vi "Rio_Trapazodial_Velocity_V2.vi"() -> ()   [LabVIEW 2017]
uses:
  <vilib>/myRIO/Common/Instrument Driver Framework/myRIO v1.0/Encoder/typedefs/Encoder Signal Mode.ctl
  <vilib>/myRIO/Instrument Drivers/Onboard IO/Encoder/typedefs/Encoder Reference.ctl
  <vilib>/myRIO/Common/Instrument Driver Framework/Utilities/typedefs/myRIO Generic Hardware Reference.ctl
  <vilib>/myRIO/Common/Instrument Driver Framework/Utilities/typedefs/Hardware Version Enum.ctl
  <vilib>/myRIO/Common/Instrument Driver Framework/Utilities/typedefs/myRIO v1.0 Reference.ctl
  <vilib>/myRIO/Common/Instrument Driver Framework/Utilities/typedefs/Generic FPGA Reference.ctl
  <vilib>/myRIO/Common/Instrument Driver Framework/myRIO v1.0/Encoder/typedefs/Encoder Channels Enum.ctl
  <vilib>/myRIO/Common/Instrument Driver Framework/myRIO v1.0/Encoder/typedefs/Encoder Configuration v1.0.ctl
  <vilib>/userdefined/High Color/nirio_resource_hc.ctl
  <vilib>/myRIO/Common/Instrument Driver Framework/Utilities/vis/Is FPGA Ref Available.vi
  <vilib>/myRIO/Common/Instrument Driver Framework/myRIO v1.0/Encoder/vis/myRIO v1.1 Open Encoder.vi
  <vilib>/myRIO/Instrument Drivers/Onboard IO/Encoder/vis/Read.vi
  <vilib>/myRIO/Common/Instrument Driver Framework/Utilities/vis/Validate Channels.vi
  <vilib>/myRIO/Common/Instrument Driver Framework/myRIO v1.0/Encoder/vis/myRIO v1.0 Reserve Encoder.vi
  <vilib>/myRIO/Common/Instrument Driver Framework/myRIO v1.0/Encoder/vis/myRIO v1.0 Build MUX Configuration Encoder.vi
  <vilib>/myRIO/Common/Instrument Driver Framework/myRIO v1.0/Resource Manager/vis/myRIO v1.0 Reserve Channel List.vi
  <vilib>/myRIO/Common/Instrument Driver Framework/myRIO v1.0/Resource Manager/vis/myRIO v1.0 Create Configuration List.vi
  <vilib>/myRIO/Common/Instrument Driver Framework/myRIO v1.0/Resource Manager/vis/myRIO v1.0 Reserve Channel.vi
  <vilib>/myRIO/Common/Instrument Driver Framework/myRIO v1.0/Resource Manager/vis/myRIO v1.0 Unreserve Channel.vi
  <vilib>/myRIO/Common/Instrument Driver Framework/myRIO v1.0/Resource Manager/vis/myRIO v1.0 Build Mutex Name.vi
  <vilib>/Utility/VariantDataType/GetNumericInfo.vi
  <vilib>/Utility/error.llb/Error Cluster From Error Code.vi
  <vilib>/myRIO/Common/Instrument Driver Framework/myRIO v1.0/myRIO v1.1 Open.vi
  <vilib>/myRIO/Common/Instrument Driver Framework/Utilities/vis/IO Manager.vi
  <vilib>/myRIO/Common/Instrument Driver Framework/Utilities/vis/Configuration Manager.vi
  <vilib>/myRIO/Common/Instrument Driver Framework/myRIO v1.0/Resource Manager/vis/myRIO v1.0 Configure IO.vi
  <vilib>/myRIO/Common/Instrument Driver Framework/myRIO v1.0/myRIO v1.0 Close.vi
  <vilib>/myRIO/Common/Instrument Driver Framework/myRIO v1.0/Encoder/vis/myRIO v1.0 Configure Encoder.vi
  <vilib>/myRIO/Common/Instrument Driver Framework/myRIO v1.0/Encoder/vis/myRIO v1.0 Read Encoder.vi
  <vilib>/addons/control/pid/pid.llb/PID (DBL).vi
  <vilib>/myRIO/Express VI/Onboard IO/Encoder/Encoder Express VI.xnode
  <vilib>/myRIO/Instrument Drivers/Onboard IO/Encoder/vis/myRIO Encoder Open.xnode
  <vilib>/myRIO/Common/Instrument Driver Framework/myRIO v1.0/Encoder/typedefs/Encoder Count Direction Enum.ctl
  <vilib>/myRIO/Instrument Drivers/Onboard IO/Encoder/Encoder.lvlib
  <vilib>/addons/control/pid/NI_PID_pid.lvlib
panel:
  out "Waveform Graph":dbl[](graph)
  in  "stop":bool
  out "element":dbl
  in  "Cluster":T1={"Start Position"=0, "End Position"=0, "Acceleration"=250}
  in  "Boolean":bool
  out "RPM Chart":dbl(graph)
  out "Counter Value":i32
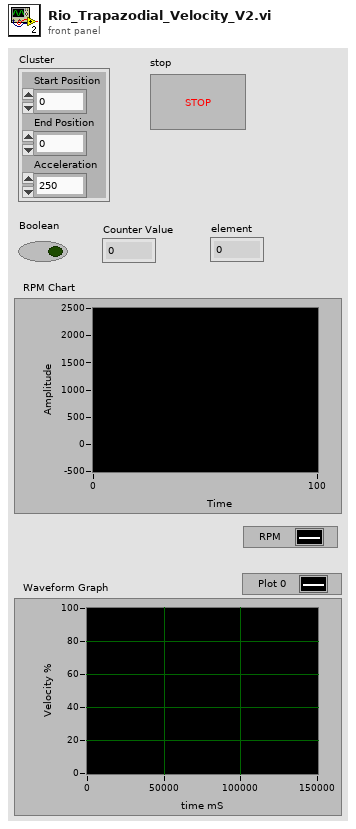
[diagram p1: front panel]
types:
  T1 = cluster{"Start Position":i64, "End Position":i64, "Acceleration":i64}
  T2 = cluster{"X(t)/Y(f) Selection ":bool, "Duty Cycle (0-1) (X Control)":dbl, "Frequency [Hz] (Y Control)":dbl, "Direction (t:+, f:-)":bool}
  T3 = cluster{"proportional gain (Kc)":dbl, "integral time (Ti, min)":dbl, "derivative time (Td, min)":dbl}
  T4 = typedef "Encoder.lvlib/Encoder Reference.ctl" = cluster{"myRIO Reference":T5, "Encoder Channels Enum":T9}
  T5 = typedef "myRIO Generic Hardware Reference.ctl" = cluster{"myRIO Model":T6, "myRIO Hardware Reference":T7}
  T6 = typedef "Hardware Version Enum.ctl" = enum16{"Unknown", "myRIO-1900", "myRIO-1950", "roboRIO", "NI ELVIS RIO CM"}
  T7 = typedef "myRIO v1.0 Reference.ctl" = cluster{"Generic FPGA Reference":T8, "Allow multiple opens":bool}
  T8 = typedef "Generic FPGA Reference.ctl" = refnum<k20>
  T9 = typedef "Encoder Channels Enum.ctl" = enum16{"Not Connected", "C/ENC0", "C/ENC1", "A/ENC", "B/ENC", "DIO/ENC0", "DIO/ENC1", "DIO/ENC2", "DIO/ENC3", "DIO/ENC4"}
  T10 = typedef "Encoder Signal Mode.ctl" = enum16{"Quadrature phase signal", "Step and direction signal"}
  T11 = typedef "nirio_resource_hc.ctl" = tag
  T12 = cluster{"Boolean":bool, dbl, dbl, "Boolean":bool}
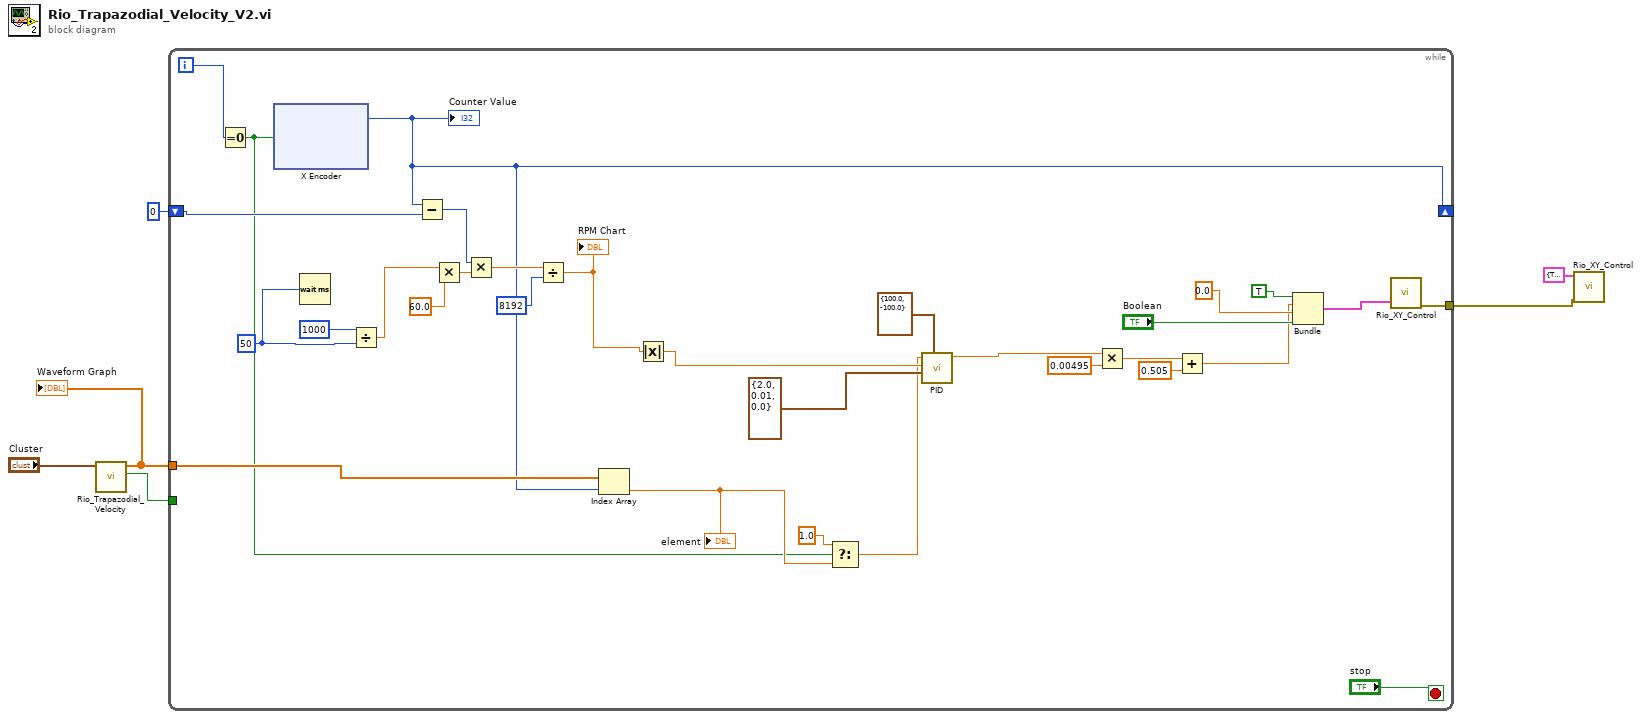
[diagram p0: block diagram]
diagram:
  n1 = call "Rio_Trapazodial_Velocity.vi"("Cluster"="Cluster") -> ("Forward (t)/Reverse (f)"=w4:bool, "Waveform Graph"=w1:dbl[])  [unwired: 8 in, 1 out]
  "Waveform Graph" <- w1
  n2 = while {
    shift-right: [w14] -> _
    shift-left: 0 ("Counter Value") -> [w17]
    tunnel: w1 -> [w15]
    tunnel: w4 -> [_]
    tunnel: [w13] -> w2
    i -> [w18]
    stop <- "stop" stop-if-true
    w27 = u32 50 ("milliseconds to wait")
    n3 = Equal To 0?(x=w18) -> (x = 0?=w9:bool)
    n4 = xnode "X Encoder"("Reset Counter"=w9) -> ("Counter Value"=w14:i32)  [unwired: 1 in, 3 out]
    "Counter Value" <- w14
    n5 = Wait (ms)(milliseconds to wait=w27) -> ()  [unwired: 1 out]
    n6 = Divide(x=u32 1000, y=w27) -> (x/y=w30:dbl)
    n7 = Subtract(x=w14, y=w17) -> (x-y=w29:i32)
    n8 = Multiply(x=w30, y=60.0) -> (x*y=w31:dbl)
    n9 = Multiply(x=w29, y=w31) -> (x*y=w28:dbl)
    n10 = Divide(x=w28, y=8192) -> (x/y=w35:dbl)
    "RPM Chart" <- w35
    n11 = Index Array(array=w15, index=w14) -> (element=w10:dbl)
    "element" <- w10
    n12 = Absolute Value(x=w35) -> (abs(x)=w36:dbl)
    n13 = Select(t=1.0, s=w9, f=w10) -> (s? t:f=w8:dbl)
    n14 = call-poly <vilib>:"PID.vi"("output range"=cluster{"output high":dbl, "output low":dbl} {"output high"=100.0, "output low"=-100.0}, "PID gains"=T3 {"proportional gain (Kc)"=2.0, "integral time (Ti, min)"=0.01, "derivative time (Td, min)"=0.0}, "process variable"=w36, "setpoint"=w8) -> ("output"=w37:dbl)  [unwired: 6 in, 1 out]
    n15 = Multiply(x=w37, y=0.00495) -> (x*y=w32:dbl)
    n16 = Add(x=w32, y=0.505) -> (x+y=w11:dbl)
    n17 = Bundle("Boolean"=TRUE, w11, 0.0, "Boolean"="Boolean") -> (w33:T12)  [unwired: 1 in]
    n18 = call "Rio_XY_Control.vi"("Input Cluster"=w33) -> ("Error Out"=w13:errorcluster)  [unwired: 10 in]
  }
  n19 = call "Rio_XY_Control.vi"("Error In"=w2, "Input Cluster"=T2 {"X(t)/Y(f) Selection "=TRUE, "Duty Cycle (0-1) (X Control)"=0.0, "Frequency [Hz] (Y Control)"=0.0, "Direction (t:+, f:-)"=TRUE}) -> ()  [unwired: 9 in, 1 out]
